vi "Get Connector Pane.vi"(8 "error in":errorcluster, 11 "VI":refnum<class "VI.lvclass">) -> (0 "error out":errorcluster, 2 "Connector Pane":picture)   [LabVIEW 2020, in "Panther Dashboard.lvlib" / "VI.lvclass"]
doc: "Get the connector pane of the vi by getting it's reference"
uses:
  VI.lvclass
  C:/GitClones/PantherDashboard/src/LabVIEW/Panther Dashboard/Class/LabVIEWItem/LabVIEWItem.lvclass
  LabVIEWItem/LabVIEWItem.lvclass/LabVIEWItem.ctl
  LabVIEWItem/Read Item Path.vi
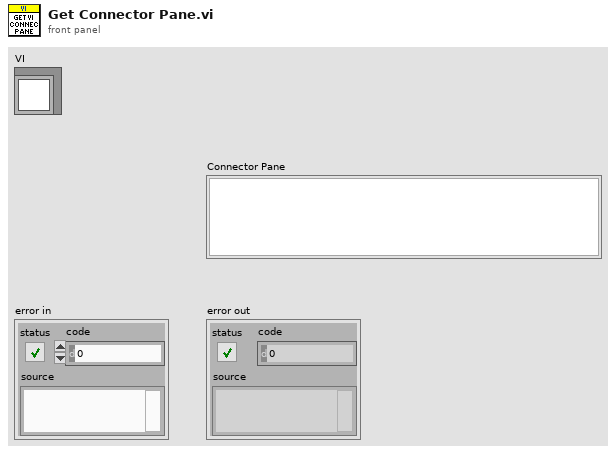
[diagram p1: front panel]
types:
  T1 = typedef "imagedata.ctl" = cluster{"image type":i32, "image depth":i32, "image":u8[], "mask":u8[], "colors":u32[], "Rectangle":cluster{"left":i16, "top":i16, "right":i16, "bottom":i16}}
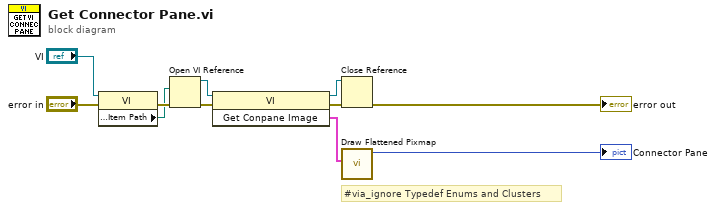
[diagram p0: block diagram]
diagram:
  # "#via_ignore Typedef Enums and Clusters"
  n1 = property class="VI"(reference="VI", error in="error in") -> (error out=w8:errorcluster, "Accessors:Item Path"=w2:path)  [unwired: 1 out]
  n2 = Open VI Reference(vi path=w2, error in (no error)=w8) -> (vi reference=w4:refnum<vi>, error out=w10:errorcluster)  [unwired: 4 in]
  n3 = invoke class="VI" method="Get Conpane Image"(reference=w4, error in=w10) -> (reference out=w1:refnum<vi>, error out=w7:errorcluster, "Get Conpane Image"=w5:T1)  [unwired: 1 in]
  n4 = Close Reference(reference=w1, error in (no error)=w7) -> (error out=→"error out":errorcluster)
  n5 = call <vilib>:"Draw Flattened Pixmap.vi"("image data"=w5) -> ("new picture"=→"Connector Pane":picture)  [unwired: 8 in]
